vi "未命名5.vi"() -> ()   [LabVIEW 2018]
panel:
  out "大小":i32
  in  "停止":bool
  out "波形图表":dbl(graph)
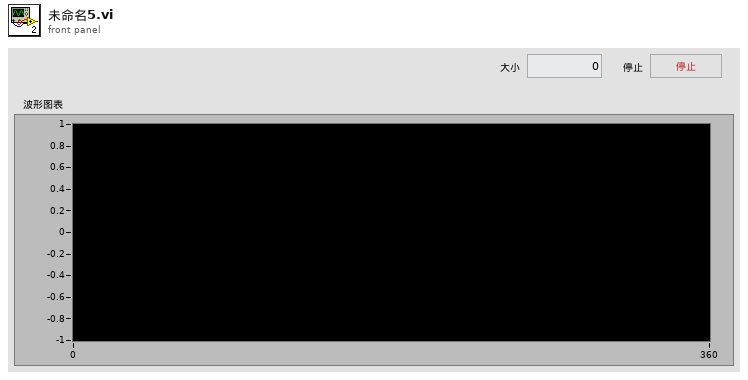
[diagram p1: front panel]
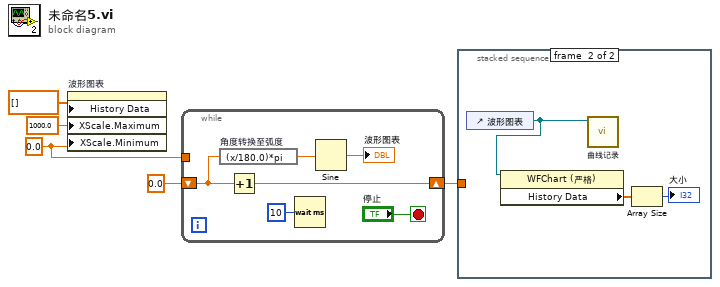
[diagram p0: block diagram]
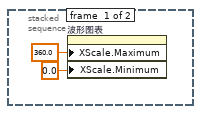
[diagram p2: hidden frame]
diagram:
  w4 = 0.0 ("X标尺.范围:最小值")
  n1 = property on="波形图表" class="WFChart (严格)"("History Data"=dbl[] [] ("历史数据"), "XScale.Maximum"=1000.0 ("X标尺.范围:最大值"), "XScale.Minimum"=w4) -> ()  [unwired: 2 in, 2 out]
  n2 = while {
    tunnel: w4 -> [_]
    shift-right: [w8] -> w1
    shift-left: 0.0 -> [w7]
    stop <- "停止" stop-if-true
    n3 = expression code="(x/180.0)*pi" "角度转换至弧度"(w7) -> (w6:dbl)
    n4 = Increment(x=w7) -> (x+1=w8:dbl)
    n5 = Wait (ms)(milliseconds to wait=u32 10 ("等待时间（毫秒）")) -> ()  [unwired: 1 out]
    n6 = Sine(x=w6) -> (sin(x)=→"波形图表":dbl)
  }
  n7 = stacked-sequence {
    tunnel: w1 -> [_ _]
    frame #0 {
      n8 = property on="波形图表" class="WFChart (严格)"("XScale.Maximum"=360.0 ("X标尺.范围:最大值"), "XScale.Minimum"=0.0 ("X标尺.范围:最小值")) -> ()  [unwired: 2 in, 2 out]
    }
    frame #1 {
      n9 = control-ref of="波形图表"() -> (w16:refnum<vi>)
      n10 = property class="WFChart (严格)"(reference=w16) -> ("History Data"=w15:dbl[])  [unwired: 1 in, 2 out]
      n11 = call "曲线记录.vi"("波形图表in"=w16) -> ()  [unwired: 11 in]
      n12 = Array Size(array=w15) -> (size(s)=→"大小":i32)
    }
  }
